vi "FABR-Create Stimulus.vi"(0 "Runtime in":T3, 2 "abort":bool, 5 "Tickets in":T1[](array[typedef]), 7 "SCL in":T2[](array[typedef]), 11 "error in (no error)":errorcluster) -> (4 "Runtime out":T3, 6 "Tickets out":T1[](array[typedef]), 8 "SCL thru":T2[](array[typedef]), 15 "error out":errorcluster)   [LabVIEW 2020]
uses:
  Typedefs/FABR-Runtime Data.ctl
  Typedefs/FABR-Stimulus Condition.ctl
  Typedefs/FABR-Stimulus Ticket.ctl
  PXI DAQ VIs/DAQ Engine VIs/PXI Globals.vi
  Utility VIs/Math VIs/dB to Linear (scalar).vi
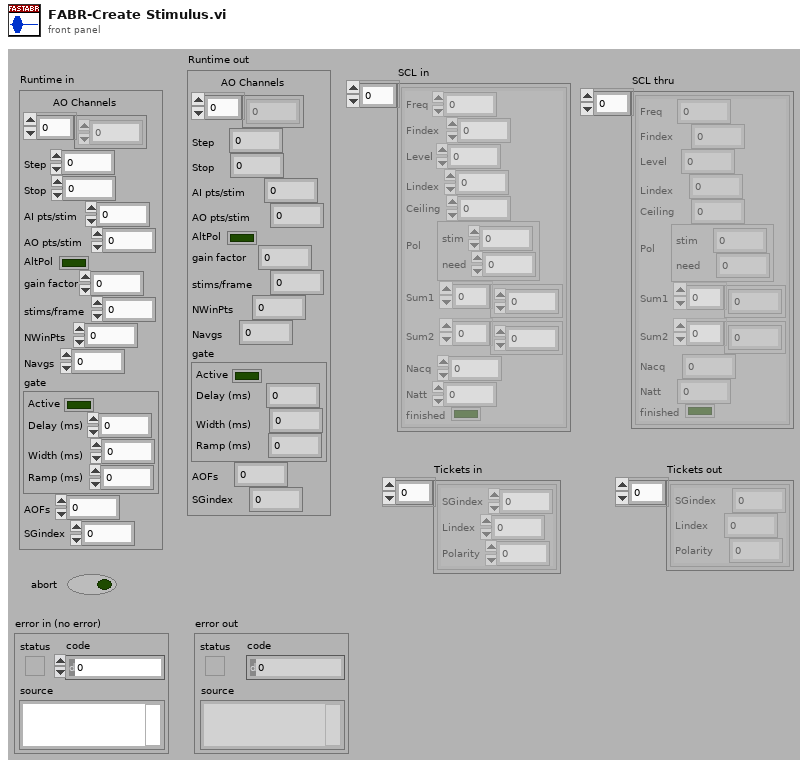
[diagram p1: front panel]
types:
  T1 = typedef "FABR-Stimulus Ticket.ctl" = cluster{"SGindex":i32, "Lindex":i32, "Polarity":i32}
  T2 = typedef "FABR-Stimulus Condition.ctl" = cluster{"Freq":dbl, "Findex":i32, "Level":dbl, "Lindex":i32, "Ceiling":dbl, "Pol":cluster{"stim":i32, "need":i32}, "Sum1":dbl[], "Sum2":dbl[], "Nacq":i32, "Natt":i32, "finished":bool}
  T3 = typedef "FABR-Runtime Data.ctl" = cluster{"AO Channels":i32[], "Step":dbl, "Stop":i32, "AI pts/stim":i32, "AO pts/stim":i32, "AltPol":bool, "gain factor":dbl, "stims/frame":i32, "NWinPts":i32, "Navgs":i32, "gate":cluster{"Active":bool, "Delay (ms)":dbl, "Width (ms)":dbl, "Ramp (ms)":dbl}, "AOFs":dbl, "SGindex":i32}
  T4 = cluster{"Active":bool, "Delay (ms)":dbl, "Width (ms)":dbl, "Ramp (ms)":dbl}
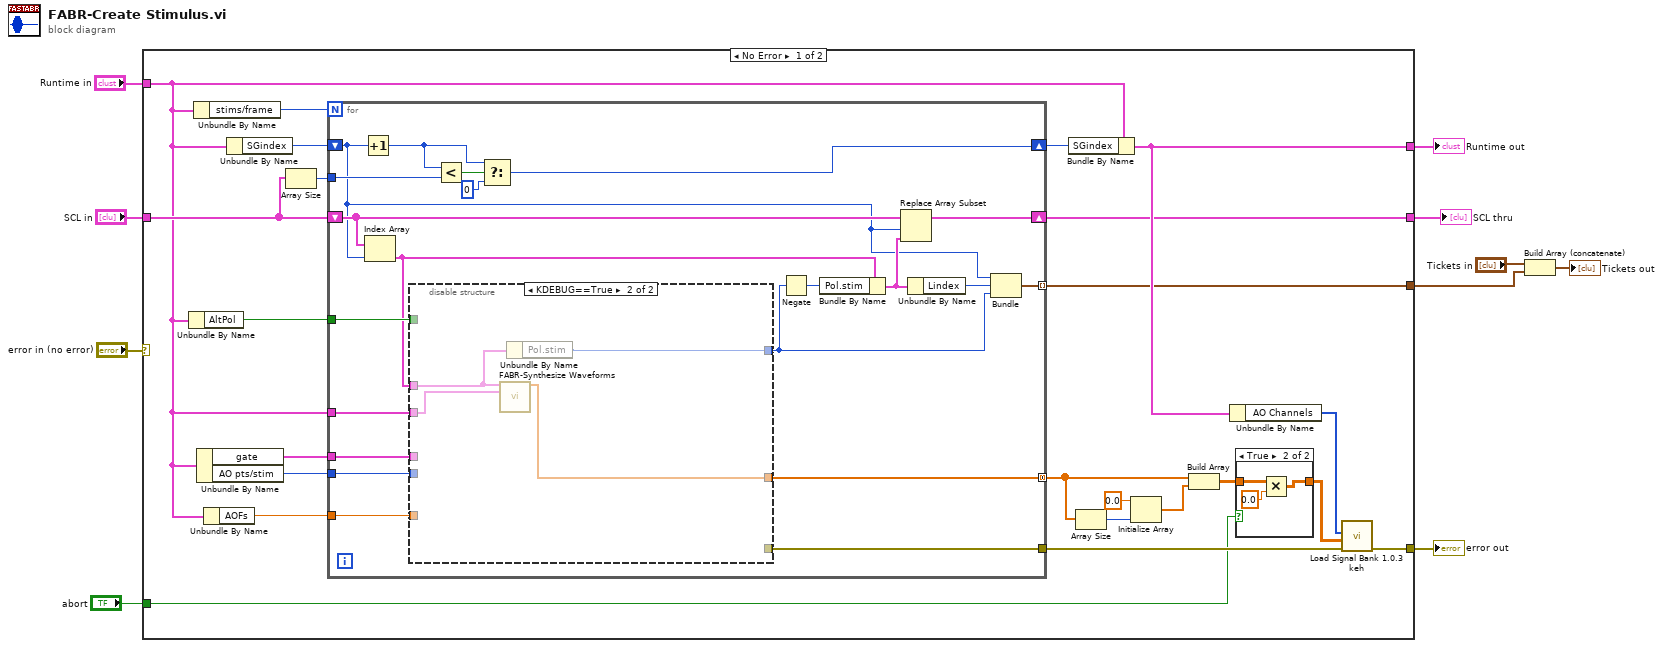
[diagram p0: block diagram]
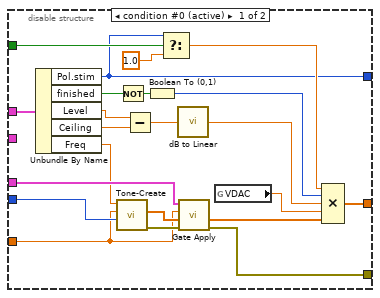
[diagram p2: hidden frame]
diagram:
  n1 = case shown="No Error" "error in (no error)" {
    selector: "error in (no error)" -> [_ w86]
    tunnel: [w19 w86] -> w10
    tunnel: "Runtime in" -> [w13 w85]
    tunnel: "SCL in" -> [w24 _]
    tunnel: [w21 w85] -> w6
    tunnel: "abort" -> [w17 _]
    tunnel: [w12 _] -> w3
    tunnel: [w11 _] -> w1
    frame No Error {
      n2 = Unbundle By Name(w13) -> ("AltPol"=w14:bool)
      n3 = Unbundle By Name(w13) -> ("stims/frame"=w28:i32)
      n4 = Unbundle By Name(w13) -> ("gate"=w30:T4, "AO pts/stim"=w31:i32)
      n5 = Unbundle By Name(w13) -> ("AOFs"=w29:dbl)
      n6 = Unbundle By Name(w13) -> ("SGindex"=w27:i32)
      n7 = Array Size(array=w24) -> (size(s)=w23:i32)
      n8 = for {
        N: w28 -> [_]
        tunnel: [w54] -> w20
        tunnel: w31 -> [w53]
        tunnel: w30 -> [w52]
        tunnel: w29 -> [w51]
        shift-right: [w46] -> w22
        shift-left: w27 -> [w34]
        tunnel: [w50] -> w25 mode=concatenating
        tunnel: w23 -> [w49]
        tunnel: w14 -> [w44]
        tunnel: w13 -> [w43]
        shift-right: [w41] -> w11
        shift-left: w24 -> [w42]
        tunnel: [w35] -> w12 mode=indexing
        n9 = Increment(x=w34) -> (x+1=w47:i32)
        n10 = Index Array(array=w42, index=w34) -> (element=w39:T2)
        n11 = disable-structure shown="KDEBUG==True" {
          disable-tunnel: [w76 _] -> w54
          disable-tunnel: w53 -> [w75 _]
          disable-tunnel: w52 -> [w70 _]
          disable-tunnel: w51 -> [w69 _]
          disable-tunnel: w39 -> [w56 w78]
          disable-tunnel: [w66 w79] -> w50
          disable-tunnel: w44 -> [w64 _]
          disable-tunnel: w43 -> [_ w80]
          disable-tunnel: [w55 w77] -> w36
          frame condition #0 (active) {
            n12 = Unbundle By Name(w56) -> ("Pol.stim"=w55:i32, "finished"=w59:bool, "Level"=w62:dbl, "Ceiling"=w61:dbl, "Freq"=w68:dbl)
            n13 = call "Tone-Create.vi"("Npts"=w75, "Sampling Rate (Hz)"=w69, "Frequency (kHz)"=w68) -> ("error out"=w74:errorcluster, "Waveform"=w73:dbl[])  [unwired: 7 in]
            n14 = Not(x=w59) -> (.not. x?=w58:bool)
            n15 = Subtract(x=w62, y=w61) -> (x-y=w60:dbl)
            n16 = Boolean To (0,1)(Boolean=w58) -> (0, 1=w65:i16)
            n17 = Select(t=w55, s=w64, f=1.0) -> (s? t:f=w63:dbl)
            n18 = call-poly "dB to Linear.vi"("dB"=w60) -> ("linear"=w67:dbl)
            n19 = call "Gate Apply.vi"("error in (no error)"=w74, "Waveform in"=w73, "Sampling Rate (Hz)"=w69, "Gate Control"=w70) -> ("error out"=w76:errorcluster, "Gated waveform"=w72:dbl[])  [unwired: 6 in]
            n20 = global read "PXI Globals.vi" "VDAC"() -> (w71:dbl)
            n21 = Compound Arithmetic op=MULTIPLY(w63, w65, w67, w71, w72) -> (w66:dbl[])
          }
          frame condition #1 {
            n22 = call "FABR-Synthesize Waveforms.vi"("SC"=w78, "Runtime in"=w80) -> ("Stim"=w79:dbl[])  [unwired: 13 in]
            n23 = Unbundle By Name(w78) -> ("Pol.stim"=w77:i32)
          }
        }
        n24 = Less?(x=w47, y=w49) -> (x < y?=w48:bool)
        n25 = Select(t=w47, s=w48, f=0) -> (s? t:f=w46:i32)
        n26 = Negate(x=w36) -> (-x=w40:i32)
        n27 = Bundle By Name(cluster=w39, "Pol.stim"=w40) -> (w38:T2)
        n28 = Replace Array Subset(array=w42, new element=w38, index=w34) -> (w41:T2[])
        n29 = Unbundle By Name(w38) -> ("Lindex"=w37:i32)
        n30 = Bundle("SGindex"=w34, "Lindex"=w37, "stim"=w36) -> (w35:cluster{"SGindex":i32, "Lindex":i32, "stim":i32})  [unwired: 1 in]
      }
      n31 = Bundle By Name(cluster=w13, "SGindex"=w22) -> (w21:T3)
      n32 = Array Size(array=w25) -> (size(s)=w26:i32)
      n33 = Initialize Array(0.0 ("element"), w26) -> (w33:dbl[])
      n34 = Build Array(w25, w33) -> (w16:dbl[][])
      n35 = Unbundle By Name(w21) -> ("AO Channels"=w18:i32[])
      n36 = case shown="True" w17 {
        tunnel: w16 -> [w81 w84]
        tunnel: [w81 w83] -> w15
        frame False {
        }
        frame True {
          n37 = Multiply(x=w84, y=0.0) -> (x*y=w83:dbl[][])
        }
      }
      n38 = call "Load Signal Bank 1.0.3 keh.vi"("error in (no error)"=w20, "Input array"=w15, "Active AO Array"=w18) -> ("error out"=w19:errorcluster)  [unwired: 6 in, 2 out]
    }
    frame Error {
    }
  }
  "error out" <- w10
  "Runtime out" <- w6
  "SCL thru" <- w1
  n39 = Build Array (concatenate)("Tickets in", w3) -> (→"Tickets out":T1[])
